vi "主程序-复材超声C扫缺陷分析评定软件.vi"() -> ()   [LabVIEW 2018]
doc: "使用该模板构建用户界面事件处理设计模式。将模板应用于对话框及其它用户界面。用户也可创建并执行VI可按照与用户界面事件相同方式处理的用户定义事件。"
uses:
  <vilib>/Utility/NIReport.llb/Report Type.ctl
  <vilib>/addons/_office/_exclsub.llb/font.ctl
  <vilib>/Utility/NIReport.llb/HTML Report Image Alignment.ctl
  <vilib>/Utility/NIReport.llb/Append Report Text (str wrap).vi
  <vilib>/Utility/NIReport.llb/Append Image to Report (path wrap).vi
  <vilib>/addons/_office/word.llb/Word Easy Table (str).vi
  <vilib>/Utility/NIReport.llb/NI_report.lvclass
  <vilib>/Utility/NIReport.llb/Word/NI_Word.lvclass
  <vilib>/addons/_office/NI_ReportGenerationToolkit.lvlib
  <vilib>/Utility/NIReport.llb/NI_ReportGenerationCore.lvlib
  <vilib>/vision/NI_Vision_Development_Module.lvlib
panel:
  out "字符串":string
  out "图像Y向分辨率（mm/像素）":dbl
  out "图像X向分辨率（mm/像素）":dbl
  out "判定为筋条的长宽比阈值":i32
  out "框号字体大小-":i16
  out "是否需要预处理":u16
  out "计入缺陷的Z值阈值":i32 caption="值"
  out "计入缺陷的面积阈值":i32
  out "报告模式":string
  in  "删除标注":bool caption="定量分析"
  out "缺陷灰度阈值":dbl caption="值"
  out "穿透图原始路径":path
  out "ROImask":T1(plugin-control)
  out "添加的路径":path
  out "连接的字符串 2":string
  out "临界面积百分比值":dbl
  out "临界Z值":i32
  out "标注后的图片路径":path
  out "全部检测结果合并":string[][](table)
  out "全部检测结果":string[][](table)
  out "部位信息":string[](array[string])=["", "34.500000", "32.500000", "1121", "34", "54.955926", "分层类", "不合格", ""]
  in  "完成标注":bool caption="定量分析"
  out "框数":dbl
  out "自定义字体":T2={"Desired Font (Application)"=enum."Application Font", "[User-specified Font]"={"Font Name"="", "Size"=12, "Strikeout?"=FALSE, "Italic?"=FALSE, "Underline?"=FALSE, "Outline?"=FALSE, "Shadow?"=FALSE, "Bold?"=FALSE, "Rotation Angle"=0.0}, "Horizontal Alignment"=0, "Vertical Alignment"=0} {"Horizontal Alignment" items=["Left", "Center", "Right"]; "Vertical Alignment" items=["Bottom", "Top", "Baseline"]}
  out "框组":T3(array[cluster])
  out "质量等级":string
  in  "stop":bool caption="停止"
  in  "导入图像":bool caption="导入图片"
  in  "开始标注":bool caption="定量分析"
  in  "查看评定结果":bool caption="辅助定性分析"
  in  "生成报告":bool caption="生成原始记录"
  in  "控件":enum32{"穿透图"}(tab)
  out "?":string
  out "穿透图":T1(plugin-control)
  out "产品规格":cluster{"产品长度（周长）（mm）":dbl, "产品宽度（母线长）（mm）":dbl}
  out "图像分辨率":T4
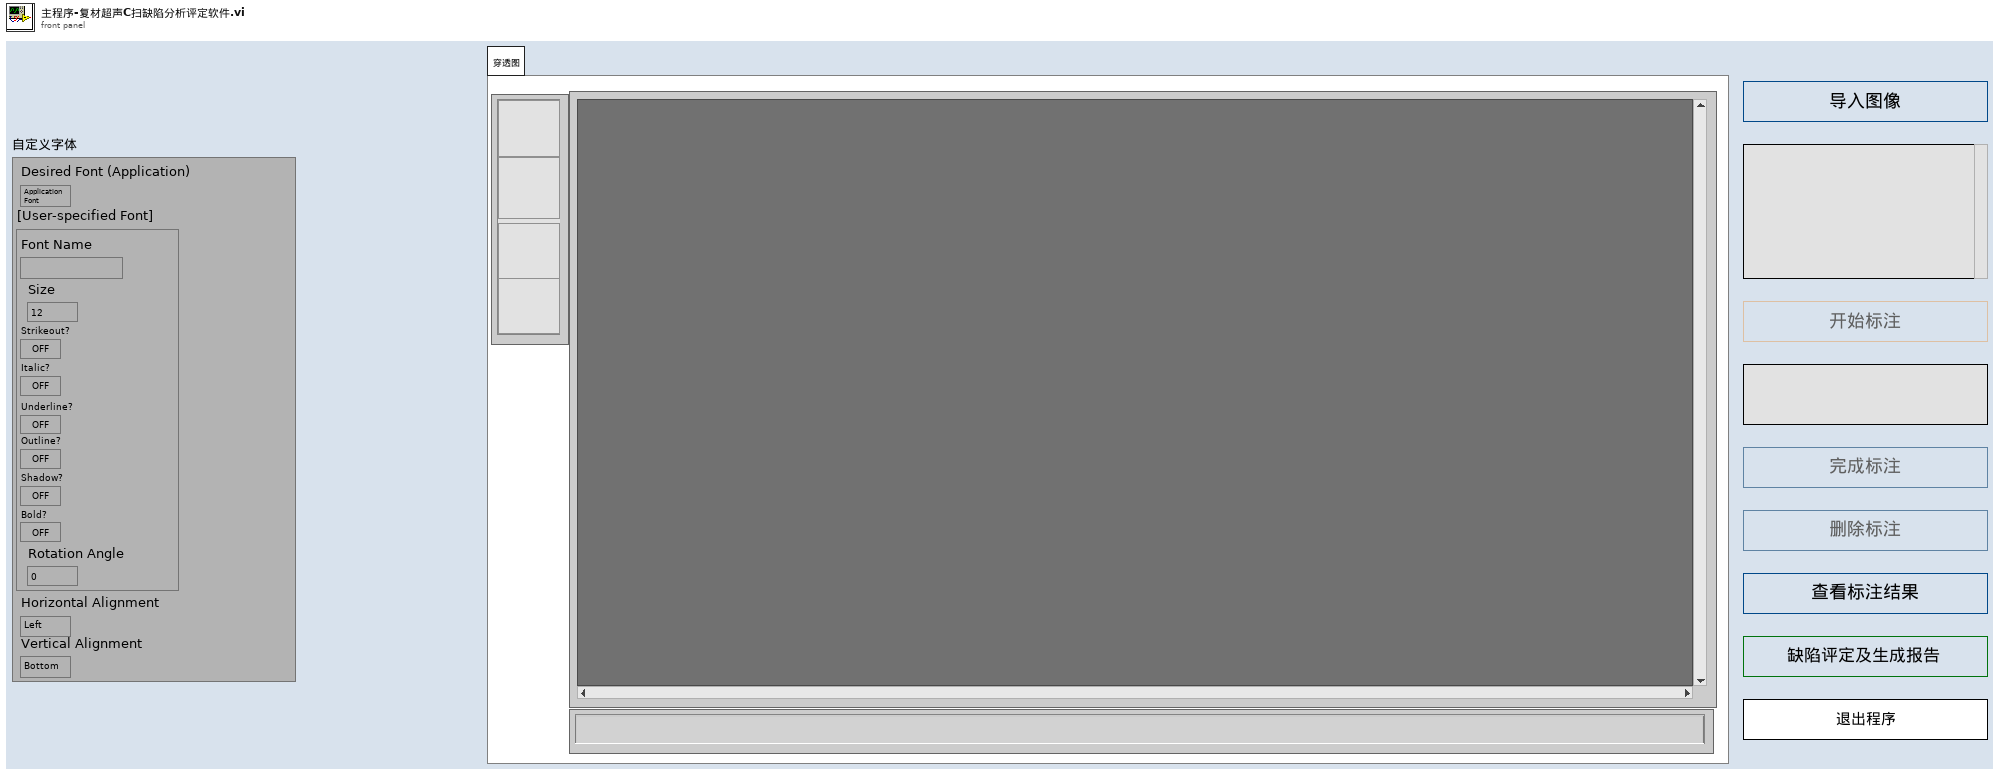
[diagram p1: front panel]
types:
  T1 = typedef "IMAQ Image.ctl" = refnum<image>
  T2 = cluster{"Desired Font (Application)":enum16{"User-specified Font", "Application Font", "System Font", "Dialog Font"}, "[User-specified Font]":cluster{"Font Name":string, "Size":i16, "Strikeout?":bool, "Italic?":bool, "Underline?":bool, "Outline?":bool, "Shadow?":bool, "Bold?":bool, "Rotation Angle":dbl}, "Horizontal Alignment":i16, "Vertical Alignment":i16}
  T3 = cluster{"Global Rectangle":i32[], "Contours":cluster{"Contour Type":u32, "ROI Type":u32, "Points":i32[]}[]}[]
  T4 = cluster{"图像X向分辨率（mm/像素）":dbl, "图像Y向分辨率（mm/像素）":dbl}
  T5 = enum8{"Enabled", "Disabled", "Disabled and Grayed Out"}
  T6 = cluster{"Global Rectangle":i32[], "Contours":cluster{"Contour Type":u32, "ROI Type":u32, "Points":i32[]}[]}
  T7 = cluster{"Zoom Tool":bool, "Selection Tool":bool, "Pan Tool":bool, "Point Tool":bool, "Line Tool":bool, "Rectangle Tool":bool, "Rotated Rectangle Tool":bool, "Polyline Tool":bool, "Polygon Tool":bool, "Freehand Tool":bool, "Closed Freehand Tool":bool, "Ellipse Tool":bool, "Annulus Tool":bool}
  T8 = enum16{"maximized", "minimized", "normal", "no change"}
  T9 = typedef "NI_ReportGenerationCore.lvlib/Report Type.ctl" = enum16{"HTML", "Word", "Excel"}
  T10 = typedef "NI_ReportGenerationCore.lvlib/HTML Report Image Alignment.ctl" = enum16{"(default)", "LEFT", "RIGHT", "TOP", "TEXTTOP", "MIDDLE", "ABSMIDDLE", "BASELINE", "BOTTOM", "ABSBOTTOM"}
  T11 = cluster{"position (Excel)":cluster{"row":i32, "column":i32}, "name (Excel)":string, "bookmark (Word)":string}
  T12 = cluster{"position (excel)":cluster{"row":i32, "column":i32}, "name (excel)":string, "bookmark (word)":string}
  T13 = typedef "NI_ReportGenerationToolkit.lvlib/font.ctl" = cluster{"font name":string, "font size":dbl, "bold":u16, "italic":u16, "underline":u16, "strike through":u16, "font color":u32}
  T14 = typedef "Image Type" = u32
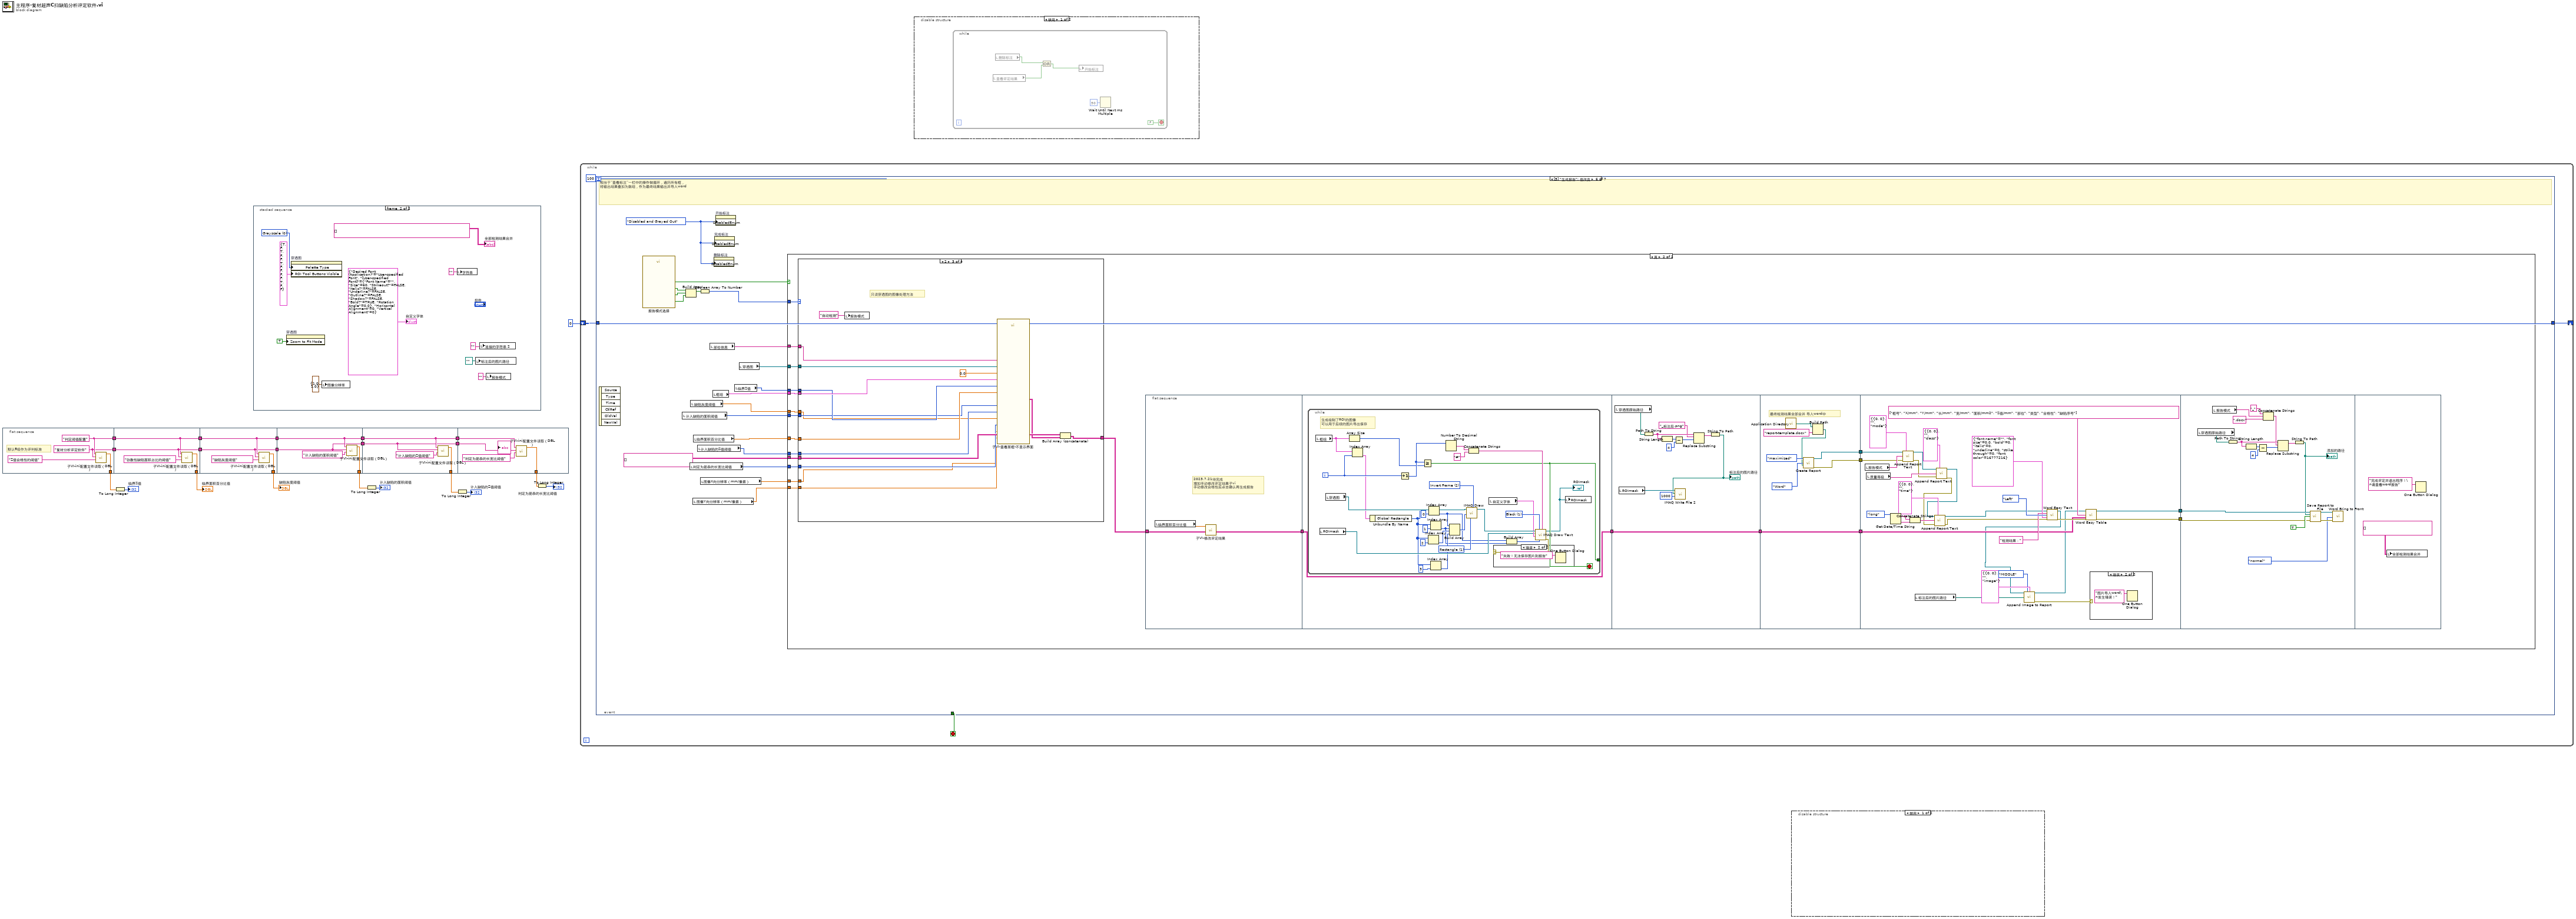
[diagram p0: block diagram]
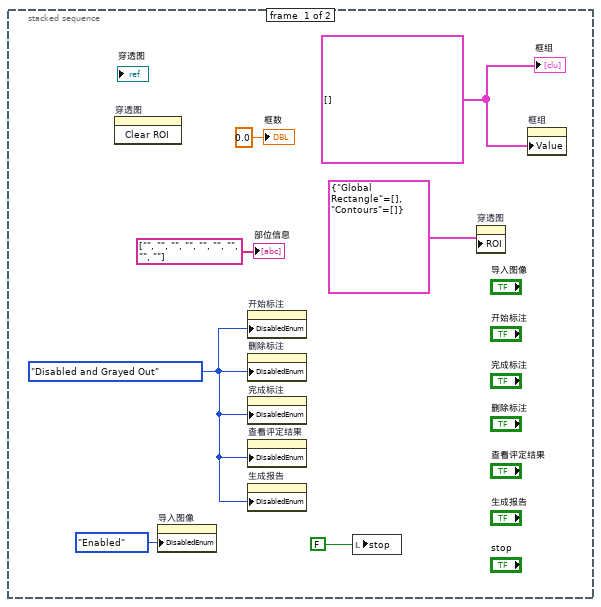
[diagram p3: hidden frame]
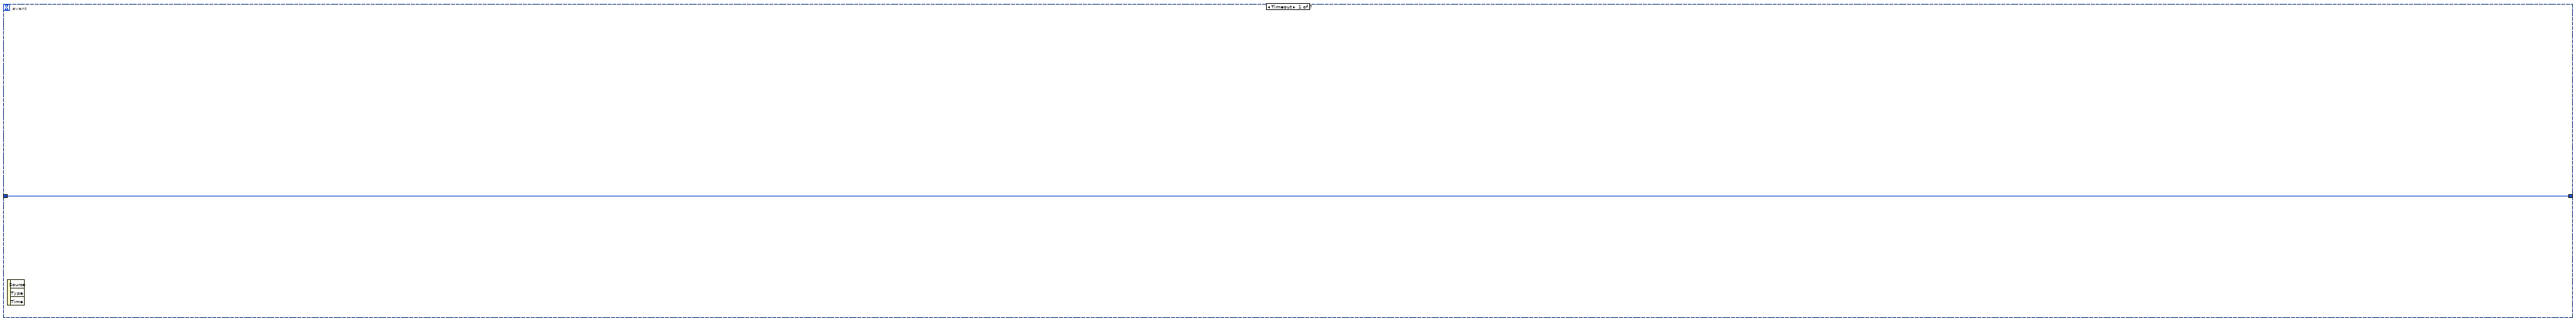
[diagram p5: hidden frame]
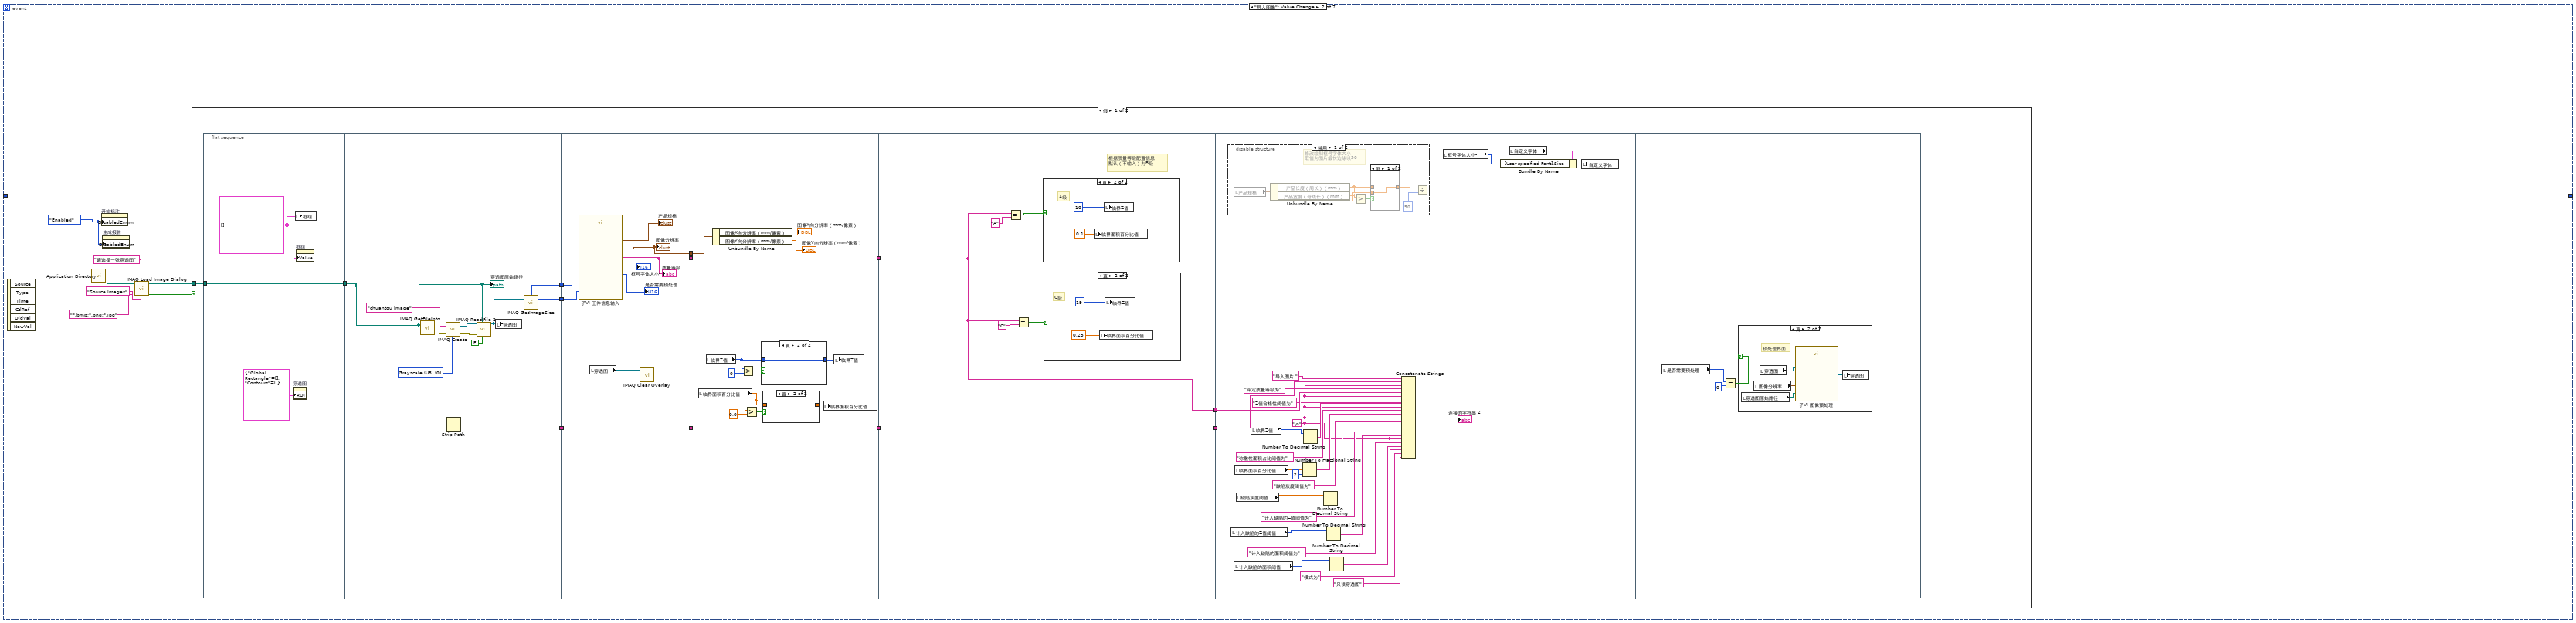
[diagram p6: hidden frame]
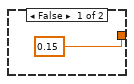
[diagram p7: hidden frame]
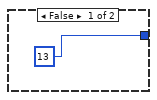
[diagram p8: hidden frame]
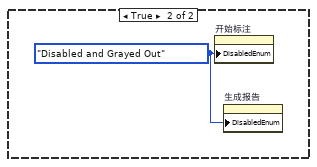
[diagram p14: hidden frame]
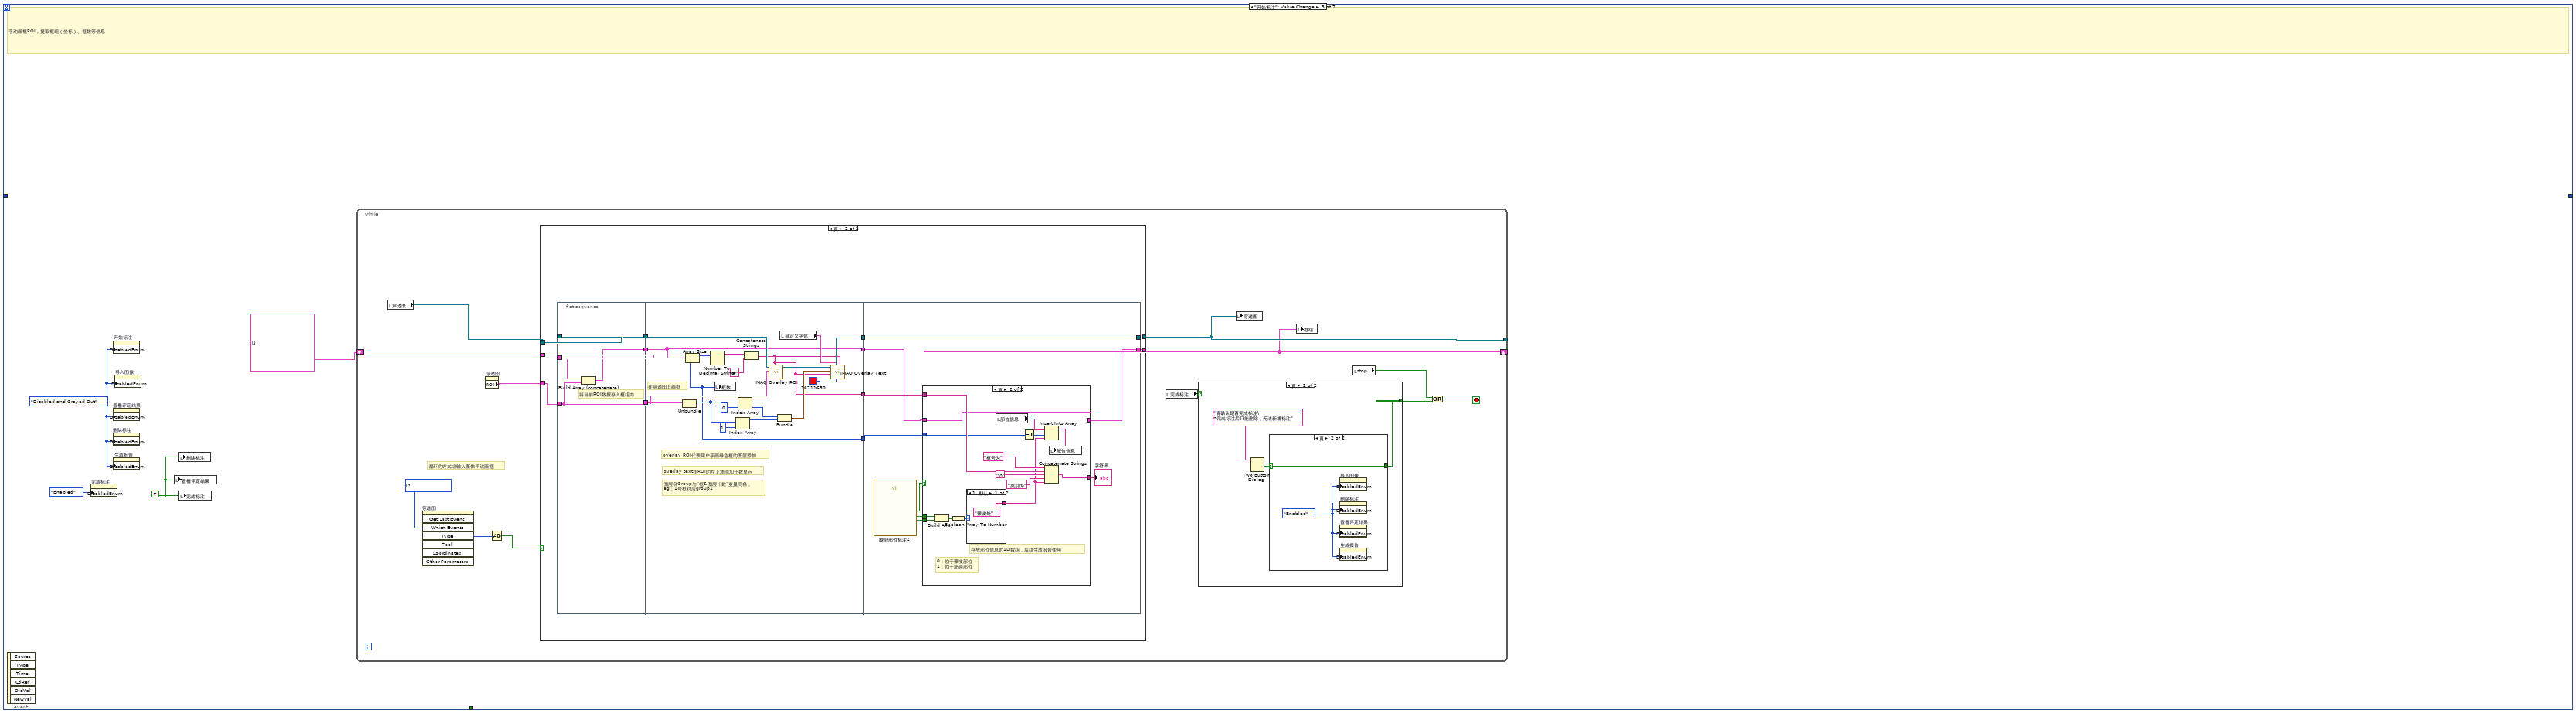
[diagram p15: hidden frame]
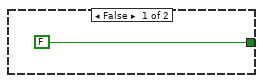
[diagram p16: hidden frame]
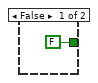
[diagram p17: hidden frame]
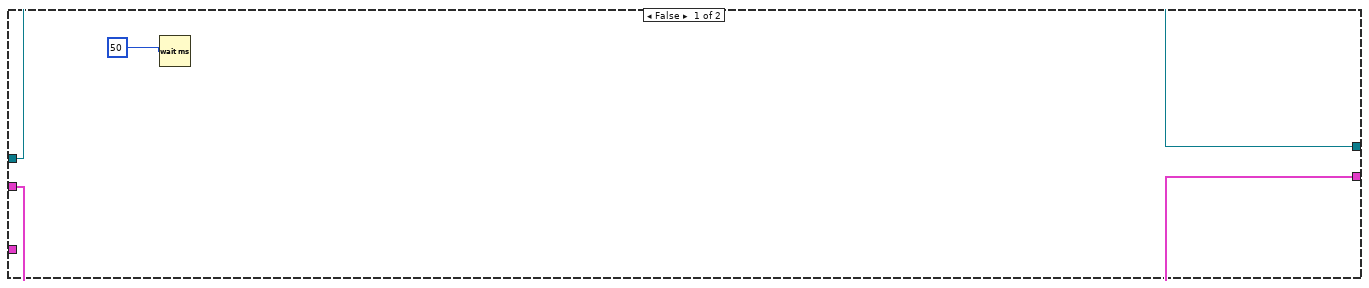
[diagram p18: hidden frame]
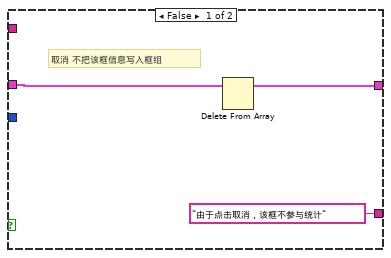
[diagram p19: hidden frame]
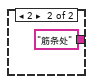
[diagram p20: hidden frame]
diagram:
  n1 = flat-sequence {
    tunnel: [w24] -> w20
    tunnel: [w23] -> w19
    tunnel: [w22] -> w14
    tunnel: w20 -> [w27]
    tunnel: w19 -> [w28]
    tunnel: [w28] -> w18
    tunnel: [w27] -> w17
    tunnel: [w26] -> w15
    tunnel: w18 -> [w30]
    tunnel: w17 -> [w31]
    tunnel: [w32] -> w16
    tunnel: [w31] -> w12
    tunnel: [w30] -> w11
    tunnel: w12 -> [w35]
    tunnel: w11 -> [w34]
    tunnel: [w36] -> w9
    tunnel: [w35] -> w8
    tunnel: [w34] -> w7
    tunnel: w8 -> [w39]
    tunnel: w7 -> [w38]
    tunnel: [w40] -> w5
    tunnel: [w39] -> w4
    tunnel: [w38] -> w3
    tunnel: w4 -> [w45]
    tunnel: w3 -> [w44]
    tunnel: [w42] -> w2
    frame #0 {
      w23 = "复材分析评定软件" ("section")
      w24 = "判定阈值配置" ("文件名称")
      # "默认B级作为评判标准"
      n2 = call "子VI-ini配置文件读取（DBL）.vi"("key"="Z值合格性的阈值", "section"=w23, "文件名称"=w24) -> ("value"=w22:dbl)  [unwired: 8 in]
    }
    frame #1 {
      n3 = call "子VI-ini配置文件读取（DBL）.vi"("key"="弥散性缺陷面积占比的阈值", "section"=w28, "文件名称"=w27) -> ("value"=w26:dbl)  [unwired: 8 in]
    }
    frame #2 {
      n4 = call "子VI-ini配置文件读取（DBL）.vi"("key"="缺陷灰度阈值", "section"=w30, "文件名称"=w31) -> ("value"=w32:dbl)  [unwired: 8 in]
    }
    frame #3 {
      n5 = call "子VI-ini配置文件读取（DBL）.vi"("key"="计入缺陷的面积阈值", "section"=w34, "文件名称"=w35) -> ("value"=w36:dbl)  [unwired: 8 in]
    }
    frame #4 {
      n6 = call "子VI-ini配置文件读取（DBL）.vi"("key"="计入缺陷的Z值阈值", "section"=w38, "文件名称"=w39) -> ("value"=w40:dbl)  [unwired: 8 in]
    }
    frame #5 {
      n7 = call "子VI-ini配置文件读取（DBL）.vi"("key"="判定为筋条的长宽比阈值", "section"=w44, "文件名称"=w45) -> ("value"=w42:dbl)  [unwired: 8 in]
    }
  }
  n8 = To Long Integer(number=w14) -> (32bit integer=→"临界Z值":i32)
  n9 = stacked-sequence {
    frame #0 {
      w50 = T3 [] ("框组")
      w47 = T5."Disabled and Grayed Out" ("禁用")
      n10 = invoke on="穿透图" class="ImageControl" method="Clear ROI"() -> ()  [unwired: 3 in, 3 out]
      n11 = property on="导入图像" class="Bool"("DisabledEnum"=T5."Enabled" ("禁用")) -> ()  [unwired: 2 in, 2 out]
      n12 = property on="开始标注" class="Bool"("DisabledEnum"=w47) -> ()  [unwired: 2 in, 2 out]
      n13 = property on="删除标注" class="Bool (严格)"("DisabledEnum"=w47) -> ()  [unwired: 2 in, 2 out]
      n14 = property on="完成标注" class="Bool (严格)"("DisabledEnum"=w47) -> ()  [unwired: 2 in, 2 out]
      n15 = property on="查看评定结果" class="Bool (严格)"("DisabledEnum"=w47) -> ()  [unwired: 2 in, 2 out]
      n16 = property on="生成报告" class="Bool"("DisabledEnum"=w47) -> ()  [unwired: 2 in, 2 out]
      n17 = local write "stop"(FALSE ("stop")) -> ()
      n18 = property on="穿透图" class="ImageControl"("ROI"=T6 {"Global Rectangle"=[], "Contours"=[]}) -> ()  [unwired: 2 in, 2 out]
      n19 = property on="框组" class="Arr (严格)"("Value"=w50) -> ()  [unwired: 2 in, 2 out]
      "部位信息" <- string[] ["", "", "", "", "", "", "", "", ""] ("部位信息")
      "框组" <- w50
      "框数" <- 0.0 ("框数")
    }
    frame #1 {
      w57 = u32 0 items=["Grayscale", "Binary", "Gradient", "Rainbow", "Temperature", "User Defined", "Binary 16 Bit", "Gradient 16 Bit", "Rainbow 16 Bit", "Temperature 16 Bit", "User Defined 16 Bit"] ("Palette:Palette Type")
      n20 = property on="穿透图" class="ImageControl"("Zoom to Fit Mode"=TRUE) -> ()  [unwired: 2 in, 2 out]
      n21 = property on="穿透图" class="ImageControl"("Palette Type"=w57, "ROI Tool Buttons Visible"=T7 {"Zoom Tool"=TRUE, "Selection Tool"=FALSE, "Pan Tool"=TRUE, "Point Tool"=FALSE, "Line Tool"=FALSE, "Rectangle Tool"=TRUE, "Rotated Rectangle Tool"=FALSE, "Polyline Tool"=FALSE, "Polygon Tool"=FALSE, "Freehand Tool"=FALSE, "Closed Freehand Tool"=TRUE, "Ellipse Tool"=FALSE, "Annulus Tool"=FALSE} ("ROI Tool Buttons Visible:All Elements")) -> ()  [unwired: 2 in, 2 out]
      n22 = local write "图像分辨率"(T4 {"图像X向分辨率（mm/像素）"=1.0, "图像Y向分辨率（mm/像素）"=1.0} ("图像分辨率")) -> ()
      n23 = local write "字符串"("" ("字符串")) -> ()
      n24 = local write "标注后的图片路径"(path "" ("标注后的图片路径")) -> ()
      n25 = local write "连接的字符串 2"("" ("连接的字符串 2")) -> ()
      n26 = local write "报告模式"("" ("报告模式")) -> ()
      "自定义字体" <- T2 {"Desired Font (Application)"=enum."User-specified Font", "[User-specified Font]"={"Font Name"="", "Size"=60, "Strikeout?"=FALSE, "Italic?"=FALSE, "Underline?"=FALSE, "Outline?"=FALSE, "Shadow?"=FALSE, "Bold?"=TRUE, "Rotation Angle"=0.0}, "Horizontal Alignment"=0, "Vertical Alignment"=0} ("Font, Size & Style")
      "全部检测结果合并" <- string[][] [] ("弥散类检测结果合并")
    }
  }
  n27 = To Long Integer(number=w9) -> (32bit integer=→"计入缺陷的面积阈值":i32)
  n28 = To Long Integer(number=w5) -> (32bit integer=→"计入缺陷的Z值阈值":i32)
  n29 = To Long Integer(number=w2) -> (32bit integer=→"判定为筋条的长宽比阈值":i32)
  n30 = while {
    shift-right: [w63] -> _
    shift-left: 0 -> [w64]
    stop <- w66 stop-if-true
    n31 = event shown="[5] \"生成报告\": 值改变" {
      selector: _ -> [_ _ _ _ _ _ _]
      dyn-events: _ -> [_ _ _ _ _ _ _]
      timeout: 100 -> [_ _ _ _ _ _ _]
      tunnel: [_ _ _ _ _ _ w552] -> w66
      tunnel: w64 -> [w67 _ _ _ _ w334 _]
      tunnel: [w67 _ _ _ _ w334 0] -> w63
      event Timeout {
        n32 = event-data() -> ()  [unwired: 1 in, 3 out]
      }
      event "导入图像": Value Change {
        w69 = T5."Enabled" ("禁用")
        n33 = event-data() -> ()  [unwired: 1 in, 6 out]
        n34 = call <vilib>:"Application Directory.vi"() -> ("Application Directory"=w68:path)
        n35 = property on="开始标注" class="Bool"("DisabledEnum"=w69) -> ()  [unwired: 2 in, 2 out]
        n36 = property on="生成报告" class="Bool"("DisabledEnum"=w69) -> ()  [unwired: 2 in, 2 out]
        n37 = call "IMAQ Load Image Dialog"("Pattern Label"="Source Images", "Prompt"="请选择一张穿透图" ("prompt"), "Pattern"="*.bmp;*.png;*.jpg", "Start Path"=w68) -> ("Cancelled?"=w71:bool, "Path"=w70:path)  [unwired: 5 in, 1 out]
        n38 = case shown="假" w71 {
          tunnel: w70 -> [w84 _]
          frame False {
            n39 = flat-sequence {
              tunnel: w84 -> [w87]
              tunnel: [w87] -> w83
              tunnel: w83 -> [w91]
              tunnel: [w93] -> w82
              tunnel: [w92] -> w81
              tunnel: [w90] -> w80
              tunnel: [w108] -> w86
              tunnel: w82 -> [w107]
              tunnel: w81 -> [w106]
              tunnel: w80 -> [w105]
              tunnel: [w105] -> w79
              tunnel: [w101] -> w75
              tunnel: w86 -> [w122]
              tunnel: [w122] -> w85
              tunnel: w79 -> [w121]
              tunnel: [w121] -> w78
              tunnel: w75 -> [w112]
              tunnel: w85 -> [w127]
              tunnel: w78 -> [w128]
              tunnel: [w128] -> w77
              tunnel: [w127] -> w76
              tunnel: w77 -> [w154]
              tunnel: w76 -> [w152]
              frame #0 {
                w88 = T3 [] ("框组")
                n40 = property on="穿透图" class="ImageControl"("ROI"=T6 {"Global Rectangle"=[], "Contours"=[]}) -> ()  [unwired: 2 in, 2 out]
                n41 = local write "框组"(w88) -> ()
                n42 = property on="框组" class="Arr (严格)"("Value"=w88) -> ()  [unwired: 2 in, 2 out]
              }
              frame #1 {
                w95 = T14 0 items=["Grayscale (U8)", "Grayscale (I16)", "Grayscale (SGL)", "Complex (CSG)", "RGB (U32)", "HSL (U32)", "RGB (U64)", "Grayscale (U16)"] ("Image Type")
                n43 = call "IMAQ GetFileInfo"("File Path"=w91) -> ("error out"=w98:errorcluster)  [unwired: 4 in, 6 out]
                n44 = call "IMAQ Create"("Image Name"="chuantou Image", "Image Type"=w95, "error in (no error)"=w98) -> ("New Image"=w99:T1, "error out"=w100:errorcluster)  [unwired: 2 in]
                n45 = Strip Path(path=w91) -> (name=w90:string)  [unwired: 1 out]
                n46 = call "IMAQ ReadFile 2"("Use File Path Image Type"=FALSE, "File Path"=w91, "error in (no error)"=w100, "Image"=w99) -> ("Image Out"=w97:T1)  [unwired: 3 in, 4 out]
                n47 = local write "穿透图"(w97) -> ()
                n48 = call "IMAQ GetImageSize"("Image"=w97) -> ("Y Resolution"=w92:i32, "X Resolution"=w93:i32)  [unwired: 3 in, 1 out]
                "穿透图原始路径" <- w91
              }
              frame #2 {
                n49 = call "子VI-工件信息输入.vi"("Y Resolution"=w106, "X Resolution"=w107) -> ("质量等级"=w108:string, "框号字体大小-"=→"框号字体大小-":i16, "产品规格"=→"产品规格":cluster{"产品长度（周长）（mm）":dbl, "产品宽度（母线长）（mm）":dbl}, "是否需要预处理"=→"是否需要预处理":u16, "图像分辨率"=w101:T4)  [unwired: 5 in]
                "图像分辨率" <- w101
                "质量等级" <- w108
                n50 = local read "穿透图"() -> (w104:T1)
                n51 = call "IMAQ Clear Overlay"("Image"=w104) -> ()  [unwired: 9 in, 2 out]
              }
              frame #3 {
                n52 = local read "临界面积百分比值"() -> (w113:dbl)
                n53 = local read "临界Z值"() -> (w114:i32)
                n54 = Unbundle By Name(w112) -> ("图像X向分辨率（mm/像素）"=→"图像X向分辨率（mm/像素）":dbl, "图像Y向分辨率（mm/像素）"=→"图像Y向分辨率（mm/像素）":dbl)
                n55 = Greater?(x=w114, y=0) -> (0:w119:bool)
                n56 = Greater?(x=w113, y=0.0) -> (0:w117:bool)
                n57 = case shown="真" w119 {
                  tunnel: [13 ("临界Z值") w126] -> w116
                  tunnel: w114 -> [_ w126]
                  frame False {
                  }
                  frame True {
                  }
                }
                n58 = case shown="真" w117 {
                  tunnel: [0.15 ("临界面积百分比值") w124] -> w115
                  tunnel: w113 -> [_ w124]
                  frame False {
                  }
                  frame True {
                  }
                }
                n59 = local write "临界面积百分比值"(w115) -> ()
                n60 = local write "临界Z值"(w116) -> ()
              }
              frame #4 {
                # "根据质量等级配置信息\n默认（不输入）为B级"
                n61 = Equal?(x=w127, y="A") -> (x = y?=w131:bool)
                n62 = Equal?(x=w127, y="C") -> (x = y?=w132:bool)
                n63 = case shown="真" w131 {
                  frame False {
                  }
                  frame True {
                    # "A级"
                    n64 = local write "临界面积百分比值"(0.1 ("临界面积百分比值")) -> ()
                    n65 = local write "临界Z值"(10 ("临界Z值")) -> ()
                  }
                }
                n66 = case shown="真" w132 {
                  frame False {
                  }
                  frame True {
                    # "C级"
                    n67 = local write "临界面积百分比值"(0.25 ("临界面积百分比值")) -> ()
                    n68 = local write "临界Z值"(19 ("临界Z值")) -> ()
                  }
                }
              }
              frame #5 {
                w142 = "\n"
                n69 = disable-structure shown="禁用" {
                  frame Disabled {
                    # "修改绘制框号字体大小\n取值为图片最长边除以50"
                    n70 = local read "产品规格"() -> (w165:cluster{"产品长度（周长）（mm）":dbl, "产品宽度（母线长）（mm）":dbl})
                    n71 = Unbundle By Name(w165) -> ("产品长度（周长）（mm）"=w167:dbl, "产品宽度（母线长）（mm）"=w168:dbl)
                    n72 = Greater?(x=w167, y=w168) -> (0:w166:bool)
                    n73 = case shown="假" w166 {
                      tunnel: w167 -> [_ w171]
                      tunnel: w168 -> [w170 _]
                      tunnel: [w170 w171] -> w169
                      frame False {
                      }
                      frame True {
                      }
                    }
                    n74 = Divide(x=w169, y=i8 50) -> ()  [unwired: 1 out]
                  }
                  frame Enabled {
                  }
                }
                n75 = local read "计入缺陷的Z值阈值"() -> (w148:i32)
                n76 = local read "计入缺陷的面积阈值"() -> (w145:i32)
                n77 = local read "临界面积百分比值"() -> (w160:dbl)
                n78 = local read "缺陷灰度阈值"() -> (w162:dbl)
                n79 = local read "临界Z值"() -> (w158:i32)
                n80 = Number To Fractional String(number=w160, precision (6)=i16 2 ("精度(6)")) -> (F-format string=w161:string)  [unwired: 2 in]
                n81 = Number To Decimal String(number=w158) -> (decimal integer string=w159:string)  [unwired: 1 in]
                n82 = Number To Decimal String(number=w162) -> (decimal integer string=w163:string)  [unwired: 1 in]
                n83 = Number To Decimal String(number=w148) -> (decimal integer string=w146:string)  [unwired: 1 in]
                n84 = Number To Decimal String(number=w145) -> (decimal integer string=w143:string)  [unwired: 1 in]
                n85 = Concatenate Strings("导入图片 " ("字符串"), w154, w142, "评定质量等级为" ("字符串"), w152, w142, "Z值合格性阈值为" ("字符串"), w159, w142, "弥散性面积占比阈值为" ("字符串"), w161, w142, "缺陷灰度阈值为" ("字符串"), w163, w142, "计入缺陷的Z值阈值为" ("字符串"), w146, w142, "计入缺陷的面积阈值为" ("字符串"), w143, w142, "模式为" ("字符串"), "只读穿透图" ("字符串")) -> (→"连接的字符串 2":string)
                n86 = local read "框号字体大小-"() -> (w138:i16)
                n87 = local read "自定义字体"() -> (w139:T2)
                n88 = Bundle By Name(cluster=w139, "[User-specified Font].Size"=w138) -> (w140:T2)
                n89 = local write "自定义字体"(w140) -> ()
              }
              frame #6 {
                n90 = local read "是否需要预处理"() -> (w173:u16)
                n91 = Equal?(x=w173, y=u16 0) -> (x = y?=w174:bool)
                n92 = case shown="真" w174 {
                  frame False {
                  }
                  frame True {
                    # "预处理界面"
                    n93 = local read "穿透图原始路径"() -> (w175:path)
                    n94 = local read "图像分辨率"() -> (w176:T4)
                    n95 = local read "穿透图"() -> (w178:T1)
                    n96 = call "子VI-图像预处理.vi"("图像分辨率"=w176, "穿透图"=w178, "穿透图原始路径"=w175) -> ("穿透图out"=w177:T1)  [unwired: 8 in]
                    n97 = local write "穿透图"(w177) -> ()
                  }
                }
              }
            }
          }
          frame True {
            w179 = T5."Disabled and Grayed Out" ("禁用")
            n98 = property on="开始标注" class="Bool"("DisabledEnum"=w179) -> ()  [unwired: 2 in, 2 out]
            n99 = property on="生成报告" class="Bool"("DisabledEnum"=w179) -> ()  [unwired: 2 in, 2 out]
          }
        }
      }
      event "开始标注": Value Change {
        w181 = T5."Disabled and Grayed Out" ("禁用")
        w183 = FALSE ("完成标注")
        # "手动画框ROI，提取框组（坐标）、框数等信息"
        n100 = event-data() -> ()  [unwired: 1 in, 6 out]
        n101 = property on="完成标注" class="Bool (严格)"("DisabledEnum"=T5."Enabled" ("禁用")) -> ()  [unwired: 2 in, 2 out]
        n102 = property on="查看评定结果" class="Bool (严格)"("DisabledEnum"=w181) -> ()  [unwired: 2 in, 2 out]
        n103 = property on="删除标注" class="Bool (严格)"("DisabledEnum"=w181) -> ()  [unwired: 2 in, 2 out]
        n104 = property on="生成报告" class="Bool"("DisabledEnum"=w181) -> ()  [unwired: 2 in, 2 out]
        n105 = property on="开始标注" class="Bool"("DisabledEnum"=w181) -> ()  [unwired: 2 in, 2 out]
        n106 = property on="导入图像" class="Bool"("DisabledEnum"=w181) -> ()  [unwired: 2 in, 2 out]
        n107 = local write "查看评定结果"(w183) -> ()
        n108 = local write "删除标注"(w183) -> ()
        n109 = local write "完成标注"(w183) -> ()
        n110 = while {
          shift-right: [w185] -> _
          shift-left: T3 [] ("框组") -> [w195]
          tunnel: [w193] -> _
          stop <- w184 stop-if-true
          (unwired) "_" ("名称或相对路径")
          (unwired) ".docx" ("名称或相对路径")
          w191 = i32[] [2] items=["No Event"=0, "Click Event"=1, "Draw Event"=2, "Size Event"=4, "Scroll Event"=5, "Double Click Event"=8] ("Which Events")
          # "循环的方式给输入图像手动画框"
          n111 = local read "穿透图"() -> (w194:T1)
          n112 = invoke on="穿透图" class="ImageControl" method="Get Last Event"("Which Events"=w191) -> ("Type"=w187:i32)  [unwired: 7 in, 7 out]
          n113 = property on="穿透图" class="ImageControl"() -> ("ROI"=w189:T6)  [unwired: 2 in, 2 out]
          n114 = Not Equal To 0?(x=w187) -> (x != 0?=w186:bool)
          n115 = case shown="真" w186 {
            tunnel: w194 -> [w206 w218]
            tunnel: [w206 w217] -> w193
            tunnel: [w204 w215] -> w185
            tunnel: w195 -> [w204 w216]
            tunnel: w189 -> [_ w214]
            frame False {
              n116 = Wait (ms)(milliseconds to wait=u32 50 ("毫秒倍数")) -> ()  [unwired: 1 out]
              n117 = Wait (ms)(milliseconds to wait=u32 50) -> ()  [unwired: 1 out]
            }
            frame True {
              n118 = flat-sequence {
                tunnel: w218 -> [w219]
                tunnel: [w219] -> w213
                tunnel: w214 -> [w222]
                tunnel: [w222] -> w212
                tunnel: w216 -> [w221]
                tunnel: [w220] -> w211
                tunnel: w213 -> [w231]
                tunnel: w212 -> [w230]
                tunnel: w211 -> [w223]
                tunnel: [w233] -> w210
                tunnel: [w223] -> w209
                tunnel: [w227] -> w208
                tunnel: [w225] -> w207
                tunnel: w210 -> [w248]
                tunnel: w209 -> [w242]
                tunnel: w208 -> [w245]
                tunnel: w207 -> [w244]
                tunnel: [w248] -> w217
                tunnel: [w241] -> w215
                frame #0 {
                  # "将当前ROI数据存入框组内"
                  n119 = Build Array (concatenate)(w221, w222) -> (w220:T3)
                }
                frame #1 {
                  # "在穿透图上画框"
                  # "图层名Group与“框&图层计数”变量同名，\neg：1号框对应group1"
                  # "overlay text在ROI的左上角添加计数显示"
                  # "overlay ROI代表用户手画绿色框的图层添加"
                  n120 = Unbundle(w230) -> ("Global Rectangle"=w238:i32[])  [unwired: 1 out]
                  n121 = Array Size(array=w223) -> (size(s)=w225:i32)
                  n122 = Number To Decimal String(number=w225) -> (decimal integer string=w226:string)  [unwired: 1 in]
                  n123 = local write "框数"(w225) -> ()
                  n124 = Index Array(array=w238, index=1 ("索引")) -> (element=w236:i32)
                  n125 = Index Array(array=w238, index=0 ("索引")) -> (element=w237:i32)
                  n126 = Concatenate Strings(w226, "#" ("字符串")) -> (w227:string)
                  n127 = call "IMAQ Overlay ROI"("Group"=w227, "ROI Descriptor"=w230, "Image"=w231) -> ("Image Out"=w239:T1)  [unwired: 7 in, 1 out]
                  n128 = Bundle(w237, w236) -> (w232:cluster{i32, i32})  [unwired: 1 in]
                  n129 = local read "自定义字体"() -> (w229:T2)
                  n130 = call "IMAQ Overlay Text"("Group"=w227, "Text Color (black)"=u32 16711680, "Font, Size & Style"=w229, "String"=w227, "Origin"=w232, "Image"=w239) -> ("Image Out"=w233:T1)  [unwired: 4 in, 1 out]
                }
                frame #2 {
                  n131 = call "缺陷部位标注2"() -> ("位于筋条处"=w247:bool, "位于蒙皮处"=w246:bool, "确定"=w243:bool)  [unwired: 16 in, 1 out]
                  n132 = case shown="真" w243 {
                    tunnel: w247 -> [_ w264]
                    tunnel: w246 -> [_ w263]
                    tunnel: w245 -> [_ w259]
                    tunnel: w244 -> [_ w256]
                    tunnel: w242 -> [w251 w253]
                    tunnel: [w250 w253] -> w241
                    tunnel: ["由于点击取消，该框不参与统计" w252] -> w240
                    frame False {
                      # "取消 不把该框信息写入框组"
                      n133 = Delete From Array(array=w251) -> (array with subset deleted=w250:T3)  [unwired: 2 in, 1 out]
                    }
                    frame True {
                      # "0：位于蒙皮部位\n1：位于筋条部位"
                      # "存放部位信息的1D数组，后续生成报告使用"
                      n134 = Build Array(w263, w264) -> (w265:bool[])
                      n135 = Boolean Array To Number(Boolean array=w265) -> (number=w266:u32)
                      n136 = case shown="1, 默认" w266 {
                        tunnel: ["蒙皮处" ("t") "筋条处" ("t")] -> w254
                        frame 1, Default {
                        }
                        frame 2 {
                        }
                      }
                      n137 = local read "部位信息"() -> (w258:string[])
                      n138 = Decrement(x=w256) -> (x-1=w255:i32)
                      n139 = Insert Into Array(array=w258, index=w255, new element=w254) -> (w257:string[])
                      n140 = Concatenate Strings("框号为" ("字符串"), w259, "\n", "类别为" ("字符串"), w254) -> (w252:string)
                      n141 = local write "部位信息"(w257) -> ()
                    }
                  }
                  "字符串" <- w240
                }
              }
            }
          }
          n142 = local read "完成标注"() -> (w190:bool)
          n143 = case shown="真" w190 {
            tunnel: [FALSE ("T button?") w197] -> w188
            frame False {
            }
            frame True {
              n144 = Two Button Dialog(message="请确认是否完成标注\n完成标注后只能删除，无法新增标注" ("消息")) -> (T button?=w198:bool)  [unwired: 2 in]
              n145 = case shown="真" w198 {
                selector: w198 -> [_ w202]
                tunnel: [FALSE w202] -> w197
                frame False {
                }
                frame True {
                  w201 = T5."Enabled" ("禁用")
                  n146 = property on="导入图像" class="Bool"("DisabledEnum"=w201) -> ()  [unwired: 2 in, 2 out]
                  n147 = property on="删除标注" class="Bool (严格)"("DisabledEnum"=w201) -> ()  [unwired: 2 in, 2 out]
                  n148 = property on="查看评定结果" class="Bool (严格)"("DisabledEnum"=w201) -> ()  [unwired: 2 in, 2 out]
                  n149 = property on="生成报告" class="Bool"("DisabledEnum"=w201) -> ()  [unwired: 2 in, 2 out]
                }
              }
            }
          }
          n150 = local write "穿透图"(w193) -> ()
          n151 = local write "框组"(w185) -> ()
          n152 = local read "stop"() -> (w192:bool)
          n153 = Or(x=w192, y=w188) -> (x .or. y?=w184:bool)
          n154 = call <vilib>:"Application Directory.vi"() -> ()  [unwired: 1 out]
        }
      }
      event "删除标注": Value Change {
        w270 = T5."Disabled and Grayed Out" ("禁用")
        n155 = event-data() -> ()  [unwired: 1 in, 6 out]
        n156 = call "用户输入2"() -> ("框号"=w271:dbl, "确定"=w272:bool)  [unwired: 17 in, 1 out]
        n157 = property on="生成报告" class="Bool"("DisabledEnum"=T5."Enabled" ("禁用")) -> ()  [unwired: 2 in, 2 out]
        n158 = property on="完成标注" class="Bool (严格)"("DisabledEnum"=w270) -> ()  [unwired: 2 in, 2 out]
        n159 = property on="开始标注" class="Bool"("DisabledEnum"=w270) -> ()  [unwired: 2 in, 2 out]
        n160 = case shown="真" w272 {
          tunnel: w271 -> [_ w273]
          frame False {
            # "用户取消操作"
          }
          frame True {
            n161 = stacked-sequence {
              tunnel: w273 -> [_ w280 _]
              frame #0 {
                # "1. 删除所有框"
                n162 = local read "穿透图"() -> (w274:T1)
                n163 = call "IMAQ Clear Overlay"("Image"=w274) -> ()  [unwired: 9 in, 2 out]
              }
              frame #1 {
                # "2. 删除框组中指定元素"
                n164 = local read "部位信息"() -> (w277:string[])
                n165 = local read "框组"() -> (w279:T3)
                n166 = Decrement(x=w280) -> (x-1=w276:dbl)
                n167 = Delete From Array(array=w277, index=w276) -> (array with subset deleted=w275:string[])  [unwired: 1 in, 1 out]
                n168 = Delete From Array(array=w279, index=w276) -> (array with subset deleted=w278:T3)  [unwired: 1 in, 1 out]
                n169 = local write "框组"(w278) -> ()
                n170 = local write "部位信息"(w275) -> ()
              }
              frame #2 {
                # "3. 重画所有框"
                n171 = while {
                  i -> [w293]
                  stop <- w284 stop-if-true
                  n172 = local read "框组"() -> (w288:T3)
                  n173 = local read "穿透图"() -> (w292:T1)
                  n174 = Array Size(array=w288) -> (size(s)=w289:i32)
                  n175 = Index Array(array=w288, index=w293) -> (element=w283:T6)
                  n176 = Increment(x=w293) -> (x+1=w300:i32)
                  n177 = local write "框数"(w289) -> ()
                  n178 = Greater Or Equal?(x=w300, y=w289) -> (x >= y?=w284:bool)
                  n179 = call "IMAQ Overlay ROI"("ROI Descriptor"=w283, "Image"=w292) -> ("Image Out"=w298:T1)  [unwired: 8 in, 1 out]
                  n180 = Unbundle(w283) -> ("Global Rectangle"=w290:i32[])  [unwired: 1 out]
                  n181 = Number To Decimal String(number=w300) -> (decimal integer string=w285:string)  [unwired: 1 in]
                  n182 = Index Array(array=w290, index=0 ("索引")) -> (element=w295:i32)
                  n183 = Index Array(array=w290, index=1 ("索引")) -> (element=w296:i32)
                  n184 = local read "自定义字体"() -> (w282:T2)
                  n185 = Concatenate Strings(w285, "#" ("字符串")) -> (w281:string)
                  n186 = Bundle(w295, w296) -> (w286:cluster{i32, i32})  [unwired: 1 in]
                  n187 = call "IMAQ Overlay Text"("Text Color (black)"=u32 16711680, "Font, Size & Style"=w282, "String"=w281, "Origin"=w286, "Image"=w298) -> ("Image Out"=w291:T1)  [unwired: 5 in, 1 out]
                  n188 = local write "穿透图"(w291) -> ()
                }
              }
            }
          }
        }
      }
      event "查看评定结果": Value Change {
        w309 = T5."Disabled and Grayed Out" ("禁用")
        # "只读穿透图的图像处理方法"
        # "查看指定框的详细信息，包括灰度和面积阈值分割后的结果，提取到的长宽面积等信息"
        n189 = event-data() -> ()  [unwired: 1 in, 6 out]
        n190 = property on="完成标注" class="Bool (严格)"("DisabledEnum"=w309) -> ()  [unwired: 2 in, 2 out]
        n191 = local read "判定为筋条的长宽比阈值"() -> (w304:i32)
        n192 = property on="开始标注" class="Bool"("DisabledEnum"=w309) -> ()  [unwired: 2 in, 2 out]
        n193 = local read "计入缺陷的面积阈值"() -> (w307:i32)
        n194 = local read "临界面积百分比值"() -> (w311:dbl)
        n195 = local read "计入缺陷的Z值阈值"() -> (w305:i32)
        n196 = local read "图像Y向分辨率（mm/像素）"() -> (w302:dbl)
        n197 = local read "图像X向分辨率（mm/像素）"() -> (w303:dbl)
        n198 = local read "缺陷灰度阈值"() -> (w306:dbl)
        n199 = local read "临界Z值"() -> (w312:i32)
        n200 = local read "部位信息"() -> (w314:string[])
        n201 = local read "穿透图"() -> (w301:T1)
        n202 = local read "框组"() -> (w313:T3)
        n203 = call "子VI-查看某框.vi"("输入框号（默认值0为整张图）"=0.0 ("框号"), "框组"=w313, "判定为筋条的长宽比阈值"=w304, "临界Z值"=w312, "缺陷灰度阈值"=w306, "临界面积百分比值"=w311, "计入缺陷的面积阈值"=w307, "计入缺陷的Z值阈值"=w305, 8:w301, "部位信息"=w314, "图像Y向分辨率（mm/像素）"=w302, "图像X向分辨率（mm/像素）"=w303) -> ("全部检测结果"=→"全部检测结果":string[][])  [unwired: 15 in]
      }
      event "生成报告": Value Change {
        w323 = T5."Disabled and Grayed Out" ("禁用")
        # "相当于“查看标注”一栏中的操作做循环，遍历所有框，\n将输出结果叠加为数组，作为最终结果输出并导入word"
        n204 = event-data() -> ()  [unwired: 1 in, 6 out]
        n205 = call "报告模式选择"() -> ("深度学习方法"=w322:bool, "自动检测结果"=w325:bool, "手动框选结果"=w326:bool, "确定"=w324:bool)  [unwired: 15 in, 1 out]
        n206 = local read "计入缺陷的面积阈值"() -> (w319:i32)
        n207 = Build Array(w326, w325, w322) -> (w328:bool[])
        n208 = local read "判定为筋条的长宽比阈值"() -> (w318:i32)
        n209 = local read "缺陷灰度阈值"() -> (w329:dbl)
        n210 = local read "图像Y向分辨率（mm/像素）"() -> (w316:dbl)
        n211 = local read "临界面积百分比值"() -> (w330:dbl)
        n212 = local read "计入缺陷的Z值阈值"() -> (w320:i32)
        n213 = Boolean Array To Number(Boolean array=w328) -> (number=w327:u32)
        n214 = local read "图像X向分辨率（mm/像素）"() -> (w317:dbl)
        n215 = local read "部位信息"() -> (w333:string[])
        n216 = local read "框组"() -> (w332:T3)
        n217 = property on="删除标注" class="Bool (严格)"("DisabledEnum"=w323) -> ()  [unwired: 2 in, 2 out]
        n218 = property on="完成标注" class="Bool (严格)"("DisabledEnum"=w323) -> ()  [unwired: 2 in, 2 out]
        n219 = property on="开始标注" class="Bool"("DisabledEnum"=w323) -> ()  [unwired: 2 in, 2 out]
        n220 = local read "临界Z值"() -> (w331:i32)
        n221 = local read "穿透图"() -> (w315:T1)
        n222 = case shown="真" w324 {
          tunnel: w333 -> [_ w350]
          tunnel: w332 -> [_ w349]
          tunnel: w331 -> [_ w348]
          tunnel: w330 -> [_ w347]
          tunnel: string[][] [] ("分层类检测结果合并 2") -> [_ w346]
          tunnel: w329 -> [_ w345]
          tunnel: w327 -> [_ w344]
          tunnel: w320 -> [_ w341]
          tunnel: w319 -> [_ w340]
          tunnel: w318 -> [_ w338]
          tunnel: w317 -> [_ w337]
          tunnel: w316 -> [_ w336]
          tunnel: w315 -> [_ w335]
          frame False {
          }
          frame True {
            n223 = case shown="2" w344 {
              tunnel: [w364 w394 w429 w437] -> w351
              tunnel: w350 -> [w366 w400 w433 _]
              tunnel: w349 -> [w367 w399 w432 _]
              tunnel: w348 -> [w369 w396 w431 w442]
              tunnel: w347 -> [w370 w397 w430 w439]
              tunnel: w346 -> [w371 w395 w428 w444]
              tunnel: w345 -> [w368 w398 w423 w441]
              tunnel: w341 -> [w362 w393 w424 w438]
              tunnel: w340 -> [w361 w392 w425 w440]
              tunnel: w338 -> [w360 w391 w422 w436]
              tunnel: w337 -> [w359 w390 w421 _]
              tunnel: w336 -> [w358 w389 w420 _]
              tunnel: w335 -> [w357 w388 w419 _]
              frame 0, Default {
                # "只读穿透图的图像处理方法"
                # "默认手动框选结果"
                n224 = local read "框数"() -> (w365:dbl)
                n225 = for {
                  N: w365 -> [_]
                  shift-right: [w387] -> w364
                  shift-left: w371 -> [w386]
                  tunnel: w366 -> [w383]
                  tunnel: w367 -> [w382]
                  tunnel: w370 -> [w381]
                  tunnel: w368 -> [w376]
                  tunnel: w369 -> [w380]
                  tunnel: w362 -> [w377]
                  tunnel: w361 -> [w378]
                  tunnel: w360 -> [w375]
                  tunnel: w359 -> [w374]
                  tunnel: w358 -> [w373]
                  tunnel: w357 -> [w372]
                  i -> [w385]
                  n226 = Increment(x=w385) -> (x+1=w384:i32)
                  n227 = call "子VI-查看某框-不显示界面.vi"("框号"=w384, "框组"=w382, "计入缺陷的Z值阈值"=w377, "临界Z值"=w380, "计入缺陷的面积阈值"=w378, "临界面积百分比值"=w381, "图像Y向分辨率（mm/像素）"=w373, "缺陷灰度阈值"=w376, 8:w372, "部位信息"=w383, "判定为筋条的长宽比阈值"=w375, "图像X向分辨率（mm/像素）"=w374) -> ("全部检测结果"=w379:string[][])  [unwired: 15 in]
                  n228 = Build Array (concatenate)(w386, w379) -> (w387:string[][])
                }
                "报告模式" <- "手动框选"
              }
              frame 1 {
                # "只读穿透图的图像处理方法"
                n229 = local read "框数"() -> (w401:dbl)
                n230 = local write "报告模式"("手动框选") -> ()
                n231 = for {
                  N: w401 -> [_]
                  shift-right: [w418] -> w394
                  shift-left: w395 -> [w417]
                  tunnel: w400 -> [w414]
                  tunnel: w399 -> [w413]
                  tunnel: w398 -> [w407]
                  tunnel: w397 -> [w412]
                  tunnel: w396 -> [w411]
                  tunnel: w393 -> [w408]
                  tunnel: w392 -> [w409]
                  tunnel: w391 -> [w406]
                  tunnel: w390 -> [w405]
                  tunnel: w389 -> [w404]
                  tunnel: w388 -> [w403]
                  i -> [w416]
                  n232 = Increment(x=w416) -> (x+1=w415:i32)
                  n233 = call "子VI-查看某框-不显示界面.vi"("框号"=w415, "框组"=w413, "计入缺陷的Z值阈值"=w408, "临界Z值"=w411, "计入缺陷的面积阈值"=w409, "临界面积百分比值"=w412, "图像Y向分辨率（mm/像素）"=w404, "缺陷灰度阈值"=w407, 8:w403, "部位信息"=w414, "判定为筋条的长宽比阈值"=w406, "图像X向分辨率（mm/像素）"=w405) -> ("全部检测结果"=w410:string[][])  [unwired: 15 in]
                  n234 = Build Array (concatenate)(w417, w410) -> (w418:string[][])
                }
              }
              frame 2 {
                # "只读穿透图的图像处理方法"
                n235 = local write "报告模式"("自动检测") -> ()
                n236 = call "子VI-查看某框-不显示界面.vi"("框号"=0.0, "框组"=w432, "计入缺陷的Z值阈值"=w424, "临界Z值"=w431, "计入缺陷的面积阈值"=w425, "临界面积百分比值"=w430, "图像Y向分辨率（mm/像素）"=w420, "缺陷灰度阈值"=w423, 8:w419, "部位信息"=w433, "判定为筋条的长宽比阈值"=w422, "图像X向分辨率（mm/像素）"=w421) -> ("全部检测结果"=w426:string[][])  [unwired: 15 in]
                n237 = Build Array (concatenate)(w428, w426) -> (w429:string[][])
              }
              frame 4 {
                # "深度学习方法自动检测demo"
                n238 = local read "穿透图原始路径"() -> (w435:path)
                n239 = local write "报告模式"("深度学习自动检测" ("报告模式")) -> ()
                n240 = call "子VI-深度学习自动检测.vi"("临界Z值"=w442, "判定为筋条的长宽比阈值"=w436, "临界面积百分比值"=w439, "缺陷灰度阈值"=w441, "计入缺陷的面积阈值"=w440, "穿透图原始路径"=w435, "计入缺陷的Z值阈值"=w438) -> ("全部检测结果"=w443:string[][])  [unwired: 8 in]
                n241 = Build Array (concatenate)(w443, w444) -> (w437:string[][])
              }
            }
            n242 = flat-sequence {
              tunnel: w351 -> [w448]
              tunnel: [w447] -> w339
              tunnel: [w449] -> w356
              tunnel: w339 -> [w449]
              tunnel: w356 -> [w490]
              tunnel: [w490] -> w355
              tunnel: w355 -> [w496]
              tunnel: [w496] -> w354
              tunnel: [w492] -> w343
              tunnel: [w491] -> w342
              tunnel: [w524] -> w353
              tunnel: [w523] -> w352
              tunnel: w354 -> [w517]
              tunnel: w343 -> [w514]
              tunnel: w342 -> [w513]
              tunnel: w352 -> [w542]
              tunnel: w353 -> [w543]
              frame #0 {
                # "2023.7.21待完成\n增加手动修改评定结果子vi\n手动修改合格性后点击确认再生成报告"
                n243 = local read "临界面积百分比值"() -> (w446:dbl)
                n244 = call "子VI-修改评定结果.vi"("全部检测结果"=w448, "临界面积百分比值"=w446) -> ("全部检测结果合并输出"=w447:string[][])  [unwired: 9 in]
              }
              frame #1 {
                n245 = while {
                  tunnel: [w467] -> _
                  i -> [w469]
                  stop <- w467 stop-if-true
                  w474 = 1 items=["White", "Black", "Inverted", "Black on White", "White on Black"] ("Color")
                  w476 = u16 2 items=["Frame", "Paint", "Invert Frame", "Invert Paint"] ("Draw Mode")
                  w471 = u16 1 items=["Line", "Rectangle", "Oval"] ("Shape to draw")
                  # "生成绘制了ROI的图像\n可以用于后续的图片导出保存"
                  n246 = local read "框组"() -> (w468:T3)
                  n247 = local read "ROImask"() -> (w464:T1)
                  n248 = local read "穿透图"() -> (w465:T1)
                  n249 = Array Size(array=w468) -> (size(s)=w477:i32)
                  n250 = Index Array(array=w468, index=w469) -> (element=w462:T6)
                  n251 = Unbundle By Name(w462) -> ("Global Rectangle"=w457:i32[])
                  n252 = Increment(x=w469) -> (x+1=w478:i32)
                  n253 = Greater Or Equal?(x=w478, y=w477) -> (x >= y?=w467:bool)
                  n254 = Index Array(array=w457, index=2 ("索引")) -> (element=w456:i32)
                  n255 = Index Array(array=w457, index=0 ("索引")) -> (element=w453:i32)
                  n256 = Index Array(array=w457, index=3 ("索引")) -> (element=w455:i32)
                  n257 = Index Array(array=w457, index=1 ("索引")) -> (element=w452:i32)
                  n258 = Number To Decimal String(number=w478) -> (decimal integer string=w472:string)  [unwired: 1 in]
                  n259 = Build Array(w453, w452, w456, w455) -> (w454:i32[])
                  n260 = call "IMAQ Draw"("Draw Mode"=w476, "Shape to draw"=w471, "Coordinates"=w454, "Image Src"=w465) -> ("Image Dst Out"=w475:T1)  [unwired: 6 in, 1 out]
                  n261 = Concatenate Strings(w472, "#" ("字符串")) -> (w470:string)
                  n262 = local read "自定义字体"() -> (w466:T2)
                  n263 = Build Array(w453, w452) -> (w451:i32[])
                  n264 = call "IMAQ Draw Text"("String"=w470, "Insertion Point"=w451, "Color"=w474, "Font, Size & Style"=w466, "Image Dst"=w464, "Image Src"=w475) -> ("error out"=w450:errorcluster, "Image Dst Out"=w463:T1)  [unwired: 2 in, 2 out]
                  "ROImask" <- w463
                  n265 = case shown="错误" w450 {
                    frame No Error {
                    }
                    frame Error {
                      n266 = One Button Dialog(message="失败！无法保存图片到报告" ("消息")) -> ()  [unwired: 1 in, 1 out]
                    }
                  }
                  n267 = local write "ROImask"(w463) -> ()
                }
              }
              frame #2 {
                n268 = local read "穿透图原始路径"() -> (w489:path)
                n269 = local read "ROImask"() -> (w481:T1)
                n270 = Path To String(path=w489) -> (string=w486:string)
                n271 = String Length(string=w486) -> (length=w487:i32)
                n272 = Subtract(x=w487, y=4) -> (x-y=w488:i32)
                n273 = Replace Substring(3:w488, 4:"_标注后.png" ("字符串"), 5:w486) -> (1:w485:string)  [unwired: 1 in, 1 out]
                n274 = String To Path(string=w485) -> (path=w480:path)
                "标注后的图片路径" <- w480
                n275 = call-poly "IMAQ Write File 2"("Image Quality"=u32 1000, "File Path"=w480, "Image"=w481) -> ()  [unwired: 7 in, 2 out]
              }
              frame #3 {
                # "最终检测结果全部合并 导入word中"
                n276 = call <vilib>:"Application Directory.vi"() -> ("Application Directory"=w495:path)
                n277 = Build Path(base path=w495, name or relative path="report-template.docx") -> (appended path=w493:path)
                n278 = call <vilib>:"Create Report.vi"("window state (normal)"=T8."maximized", "report type"=Report_Type."Word", "template (empty)"=w493) -> ("report out"=w492:refnum<class "NI_report.lvclass">, "error out"=w491:errorcluster)  [unwired: 11 in]
              }
              frame #4 {
                n279 = local read "报告模式"() -> (w515:string)
                n280 = local read "质量等级"() -> (w511:string)
                n281 = Get Date/Time String(date format (0)=enum16{"short", "long", "abbreviated"}."long" ("日期格式(0)")) -> (date string=w521:string, time string=w522:string)  [unwired: 2 in]
                n282 = call-poly <vilib>:"Append Report Text.vi"("report in"=w514, "MS Office parameters"=T12 {"position (excel)"={"row"=0, "column"=0}, "name (excel)"="", "bookmark (word)"="mode"}, "text"=w515, "error in (no error)"=w513) -> ("report out"=w510:refnum<class "NI_report.lvclass">, "error out"=w509:errorcluster)  [unwired: 8 in, 2 out]
                n283 = Concatenate Strings(w521, w522) -> (w520:string)
                n284 = local read "标注后的图片路径"() -> (w504:path)
                n285 = call-poly <vilib>:"Append Report Text.vi"("report in"=w510, "MS Office parameters"=T12 {"position (excel)"={"row"=0, "column"=0}, "name (excel)"="", "bookmark (word)"="class"}, "text"=w511, "error in (no error)"=w509) -> ("report out"=w507:refnum<class "NI_report.lvclass">, "error out"=w508:errorcluster)  [unwired: 8 in, 2 out]
                n286 = call-poly <vilib>:"Append Report Text.vi"("report in"=w507, "MS Office parameters"=T12 {"position (excel)"={"row"=0, "column"=0}, "name (excel)"="", "bookmark (word)"="time"}, "text"=w520, "error in (no error)"=w508) -> ("report out"=w501:refnum<class "NI_report.lvclass">, "error out"=w502:errorcluster)  [unwired: 8 in, 2 out]
                n287 = call <vilib>:"Word Easy Text.vi"("report in"=w501, "text"="检测结果：", "alignment (left)"=enum16{"Left", "Centered", "Right", "Justify"}."Left", "font"=T13 {"font name"="", "font size"=0.0, "bold"=0, "italic"=0, "underline"=0, "strike through"=0, "font color"=16777216}, "error in (no error)"=w502) -> ("report out"=w500:refnum<class "NI_report.lvclass">, "error out"=w526:errorcluster)  [unwired: 8 in, 1 out]
                n288 = call-poly <vilib>:"Append Image to Report.vi"("report in"=w500, "alignment (default)"=HTML_Report_Image_Alignment."MIDDLE", "MS Office parameters"=T11 {"position (Excel)"={"row"=0, "column"=0}, "name (Excel)"="", "bookmark (Word)"="image"}, "path or URL of image"=w504) -> ("report out"=w499:refnum<class "NI_report.lvclass">, "error out"=w503:errorcluster)  [unwired: 8 in, 2 out]
                n289 = call-poly <vilib>:"Word Easy Table.vi"("report in"=w499, "column headers"=string[] ["框号", "X/mm", "Y/mm", "长/mm", "宽/mm", "面积/mm2", "Z值/mm", "部位", "类型", "合格性", "缺陷序号"], "data"=w517, "error in (no error)"=w526) -> ("report out"=w524:refnum<class "NI_report.lvclass">, "error out"=w523:errorcluster)  [unwired: 9 in, 1 out]
                n290 = case shown="错误" w503 {
                  frame No Error {
                  }
                  frame Error {
                    n291 = One Button Dialog(message="图片导入word\n发生错误！" ("消息")) -> ()  [unwired: 1 in, 1 out]
                  }
                }
              }
              frame #5 {
                n292 = local read "穿透图原始路径"() -> (w535:path)
                n293 = local read "报告模式"() -> (w533:string)
                n294 = Path To String(path=w535) -> (string=w539:string)
                n295 = String Length(string=w539) -> (length=w540:i32)
                n296 = Subtract(x=w540, y=4) -> (x-y=w541:i32)
                n297 = Concatenate Strings("_" ("字符串"), w533, ".docx" ("字符串")) -> (w531:string)
                n298 = Replace Substring(3:w541, 4:w531, 5:w539) -> (1:w538:string)  [unwired: 1 in, 1 out]
                n299 = String To Path(string=w538) -> (path=w536:path)
                "添加的路径" <- w536
                n300 = call-dynamic "Save Report to File.vi"("report in"=w543, "report file path"=w536, "prompt to replace? (F)"=TRUE, "error in (no error)"=w542) -> ("report out"=w547:refnum<class "NI_report.lvclass">, "error out"=w546:errorcluster)  [unwired: 10 in]
                n301 = call <vilib>:"Word Bring to Front.vi"("report in"=w547, "window state (maximized)"=enum16{"maximized", "minimized", "normal"}."normal", "error in (no error)"=w546) -> ()  [unwired: 11 in, 2 out]
              }
              frame #6 {
                n302 = local write "全部检测结果合并"(string[][] [] ("弥散类检测结果合并")) -> ()
                n303 = One Button Dialog(message="完成评定并退出程序！\n请查看word报告" ("消息")) -> ()  [unwired: 1 in, 1 out]
              }
            }
          }
        }
      }
      event "stop": Value Change {
        # "退出软件"
        n304 = event-data() -> ("NewVal"=w553:bool)  [unwired: 1 in, 4 out]
        n305 = Two Button Dialog(message="是否关闭本软件？" ("消息")) -> (T button?=w554:bool)  [unwired: 2 in]
        n306 = And(x=w553, y=w554) -> (x .and. y?=w552:bool)
        n307 = case shown="真" w552 {
          frame False {
          }
          frame True {
            n308 = local read "穿透图"() -> (w556:T1)
            n309 = call "IMAQ Dispose"("All Images? (No)"=TRUE, "Image"=w556) -> ()  [unwired: 4 in, 1 out]
            n310 = disable-structure shown="RUN_TIME_ENGINE==True" {
              frame condition #0 {
                n311 = Quit LabVIEW() -> ()  [unwired: 1 in]
              }
              frame condition #1 (active) {
                n312 = Stop() -> ()  [unwired: 1 in]
              }
            }
          }
        }
      }
    }
  }
  n313 = disable-structure shown="禁用" {
    frame Disabled {
      n314 = while {
        stop <- FALSE stop-if-true
        n315 = local read "查看评定结果"() -> (w559:bool)
        n316 = local read "删除标注"() -> (w560:bool)
        n317 = Or(x=w560, y=w559) -> (x .or. y?=w561:bool)
        n318 = local write "开始标注"(w561) -> ()
        n319 = Wait Until Next ms Multiple(millisecond multiple=u32 50 ("毫秒倍数")) -> ()  [unwired: 1 out]
      }
    }
    frame Enabled {
    }
  }
  n320 = disable-structure shown="禁用" {
    frame Disabled {
    }
    frame Enabled {
    }
  }
  "临界面积百分比值" <- w15
  "缺陷灰度阈值" <- w16
